vi "ADS1015.vi"() -> ()   [LabVIEW 2014]
uses:
  <vilib>/MakerHub/LINX/Public/Utilities/Open Local.vi
  <vilib>/MakerHub/LINX/Public/Peripherals/Analog/Analog Write 1 Chan.vi
  <vilib>/MakerHub/LINX/LMH-LINX.lvlib
panel:
  out "Data":u8[](array[numeric])
  out "ADC1015":dbl(slide) scale=0.0..10.0
  in  "AO Value":dbl(slide) scale=0.0..10.0
  in  "AO Channel":u8
  in  "stop":bool
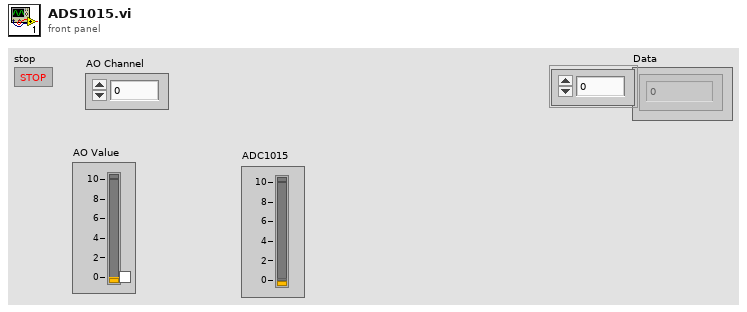
[diagram p1: front panel]
types:
  T1 = typedef "LMH-LINX.lvlib/LINX Ref.ctl" = cluster{"IO":T2, "Interface":T3, "LINX Device Config":T4}
  T2 = typedef "LMH-LINX.lvlib/Platform.ctl" = enum16{"Remote", "Local"}
  T3 = typedef "LMH-LINX.lvlib/Interface.ctl" = enum16{"Serial", "TCP"}
  T4 = typedef "LMH-LINX.lvlib/Device.lvlib/LINX Device Config.ctl" = cluster{"Interface":T3, "COM Port":refnum<visa-resource-name>, "TCP Configuration":T5, "Device Family":u8, "Device ID":u8, "Device Name":string, "TCP Ref":refnum<k5>, "Channels":T6}
  T5 = typedef "LMH-LINX.lvlib/Device.lvlib/TCP Config.ctl" = cluster{"IP Address":string, "Port":u16}
  T6 = typedef "LMH-LINX.lvlib/Channels.ctl" = cluster{"DI":u8[], "DO":u8[], "AI":u8[], "AO":u8[], "PWM":u8[], "QE":u8[], "UART":u8[], "I2C 2":u8[], "SPI":u8[], "CAN":u8[], "Servo":u8[], "AI Ref (V)":dbl, "AI Resolution (Bits)":u8, "AO Ref (V)":dbl, "AO Resolution (Bits)":u8}
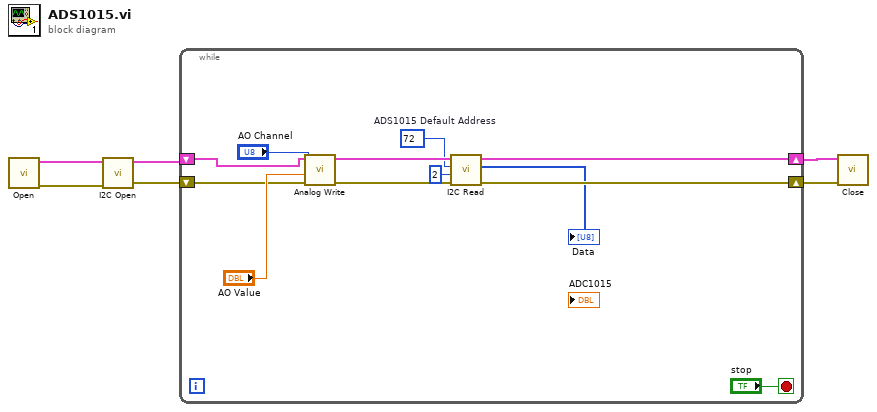
[diagram p0: block diagram]
diagram:
  n1 = call-poly <vilib>:"Open.vi"() -> ("Error Out"=w3:errorcluster, "LINX Resource"=w6:T1)  [unwired: 9 in, 1 out]
  n2 = call <vilib>:"I2C Open.vi"("Error In"=w3, "LINX Resource"=w6) -> ("Error Out"=w4:errorcluster, "LINX Resource"=w5:T1)  [unwired: 8 in]
  n3 = while {
    shift-right: [w9] -> w2
    shift-left: w5 -> [w15]
    shift-right: [w8] -> w1
    shift-left: w4 -> [w14]
    stop <- "stop" stop-if-true
    w11 = u8 72  # ADS1015 Default Address
    n4 = call-poly <vilib>:"Analog Write.vi"("Error In"=w14, "AO Value"="AO Value", "AO Channel"="AO Channel", "LINX Resource"=w15) -> ("Error Out"=w12:errorcluster, "LINX Resource"=w13:T1)  [unwired: 6 in]
    n5 = call <vilib>:"I2C Read.vi"("Error In"=w12, "Bytes To Read"=u8 2, "I2C Slave Address (0)"=w11, "LINX Resource"=w13) -> ("Error Out"=w8:errorcluster, "Data"=→"Data":u8[], "LINX Resource"=w9:T1)  [unwired: 5 in]
  }
  n6 = call <vilib>:"Close.vi"("Error In"=w1, "LINX Resource"=w2) -> ()  [unwired: 9 in, 1 out]
